vi "AES-InvCipher-BLOCK.vi"(8 "error in (no error)":errorcluster, 10 "Cipher Key":u8[](array[numeric]) format="%02x", 11 "cipher [U8]":u8[](array[numeric]) format="%02x") -> (0 "error out":errorcluster, 3 "plain [U8]":u8[](array[numeric]) format="%02x")   [LabVIEW 2020, in "Encryption.lvlib"]
doc: "Unencrypt a block of U8s that are encrypted with AES.\n\nCAUTION:\nThis VI is not secure, it does not protect the memory of the encryption, key and unencrypted data.\n\n(c) Ton Plomp, 2011\nTHIS SOFTWARE IS PROVIDED AS IS, AND ANY WARRANTY IS REJECTED"
uses:
  Encryption.lvlib
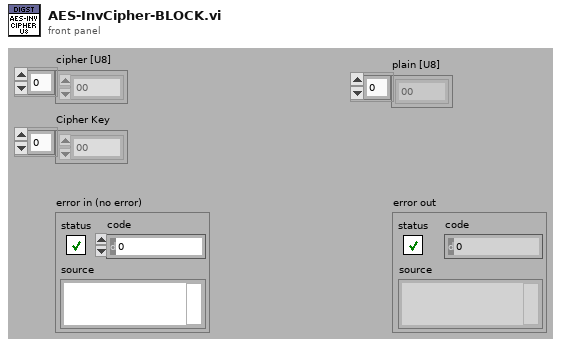
[diagram p1: front panel]
types:
  T1 = cluster{bool, i32, "String to Prepend to source (\"\")":string}
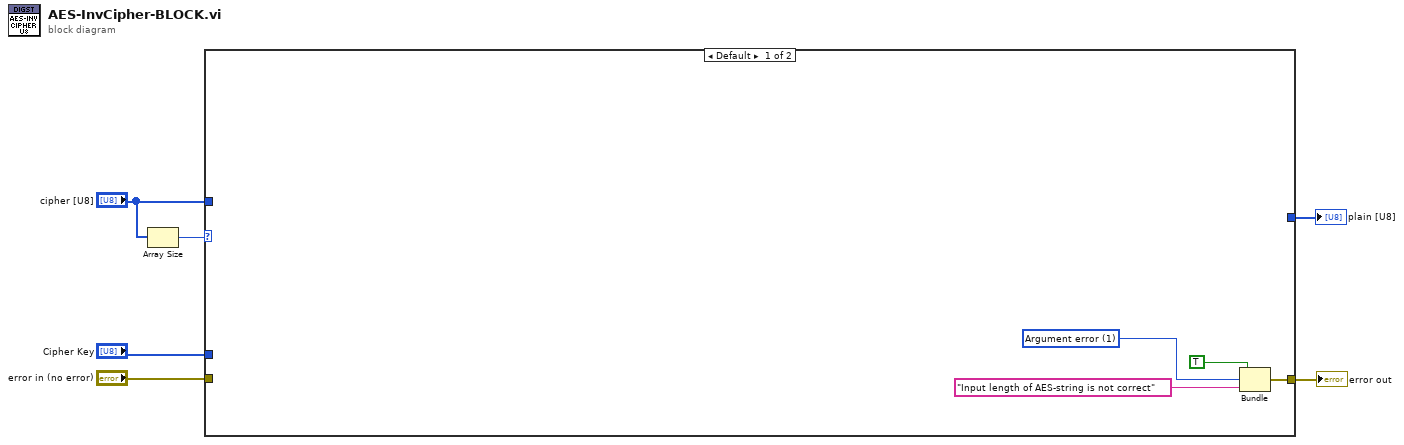
[diagram p0: block diagram]
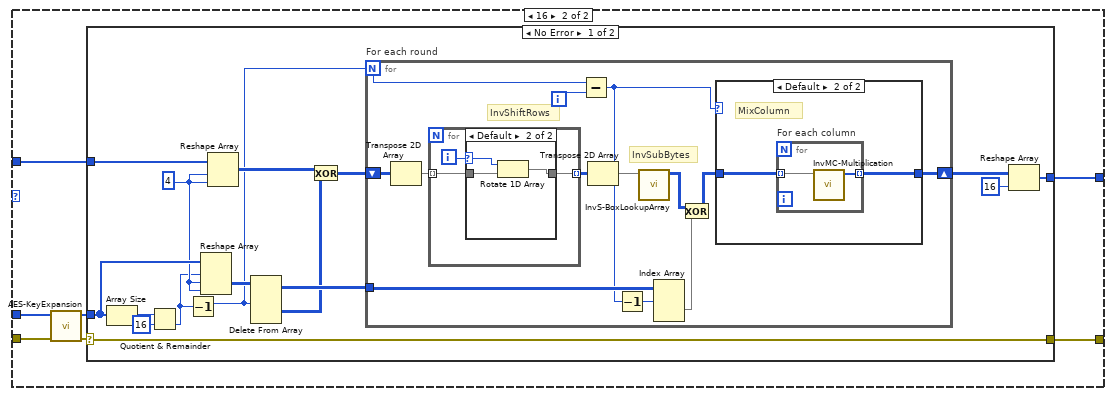
[diagram p2: hidden frame]
diagram:
  n1 = Array Size(array="cipher [U8]") -> (size(s)=w2:i32)
  n2 = case shown="Default" w2 {
    tunnel: [_ w16] -> w6
    tunnel: "Cipher Key" -> [_ w15]
    tunnel: "error in (no error)" -> [_ w14]
    tunnel: "cipher [U8]" -> [_ w13]
    tunnel: [w7 w11] -> w1
    frame Default {
      w8 = 1 items=["No error", "Argument error", "Memory is full", "Out of zone", "End of file", "File already open", "Generic file I/O error", "File not found", "File permission error", "Disk is full", "Duplicate path", "Too many files open", "System feature not enabled", "Resource file not found", "Cannot add resource", "Resource not found", "Image not found", "Image memory error", "Pen does not exist", "Config type invalid", "Config token not found", "Config parse error", "Config memory error", "Bad external code format", "Bad external code offset", "External code not present", "Null window", "Destroy window error", "Null menu", "Print aborted", "Bad print record", "Print driver error", "Windows error during printing", "Memory error during printing", "Print dialog error", "Generic print error", "Invalid device refnum", "Device not found", "Device parameter error", "Device unit error", "Cannot open device", "Device call aborted", "Generic error", "Cancelled by user", "Object ID too low", "Object ID too high", "Object not in heap", "Unknown heap", "Unknown object (invalid DefProc)", "Unknown object (DefProc not in table)", "Message out of range", "Invalid (null) method", "Unknown message", "Manager call not supported", "Bad address", "Network operation in progress", "Network operation timed out", "Connection is busy", "Network attribute not supported", "Network error", "Address in use", "System out of memory", "Connection aborted", "Connection refused", "Not connected", "Already connected", "Connection closed", "Initialization error (interapplication manager)", "Bad occurrence", "Wait on unbound occurrence handler", "Occurrence queue overflow", "Datalog type conflict", "Unused", "Unrecognized type (interapplication manager)", "Memory corrupt", "Failed to make temporary DLL", "Old CIN version", "Drag socket not found", "Failed to load drop-object", "Failed to register OLE object", "Failed to release OLE object", "Format specifier type mismatch", "Unknown format specifier", "Too few format specifiers", "Too many format specifiers", "Scan failed", "Newer CIN version", "Error converting to variant", "Runtime menu error", "Password tampered", "Variant attribute not found", "Incompatible variant data type", "Event data is not available", "Event Store is not present", "Occurrence is not found", "Event Queue is not created", "Event info is not available", "Refnum passed is NULL", "Error retrieving Class GUID", "Error retrieving CoClass GUID", "Error retrieving TypeLib GUID.", "Bad built application magic bytes.", "Specific driver is different from the specific driver associated with the Logical Name.", "There is no session opened to the class driver.", "Max Error", "MAX - Error with config objects", "MAX - Error loading configuration", "MAX - Group not supported"]
      n3 = Bundle(TRUE, w8, "String to Prepend to source (\"\")"="Input length of AES-string is not correct" ("String to Prepend to source (\"\")")) -> (w7:T1)  [unwired: 1 in]
    }
    frame 16 {
      n4 = call "AES-KeyExpansion.vi"("error in (no error)"=w14, "Key In"=w15) -> ("error out"=w12:errorcluster, "Expanded Key [U8]"=w17:u8[])  [unwired: 8 in]
      n5 = case shown="No Error" w12 {
        selector: w12 -> [w22 w59]
        tunnel: w17 -> [w31 _]
        tunnel: [w26 _] -> w16
        tunnel: w13 -> [w24 _]
        tunnel: [w22 w59] -> w11
        frame No Error {
          w23 = 4 ("y")
          n6 = Array Size(array=w31) -> (size(s)=w33:i32)
          n7 = Quotient & Remainder(x=w33, y=16) -> (floor(x/y)=w19:i32)  [unwired: 1 out]
          n8 = Decrement(x=w19) -> (x-1=w18:i32)
          n9 = Reshape Array(w31, w19, w23, w23) -> (w30:u8[][][])
          n10 = Reshape Array(w24, w23, w23) -> (w21:u8[][])
          n11 = Delete From Array(array=w30, index (dim 0)=w18) -> (deleted portion=w20:u8[][], array with subset deleted=w29:u8[][][])  [unwired: 3 in]
          n12 = Exclusive Or(1:w20, 2:w21) -> (0:w28:u8[][])
          n13 = for "For each round" {
            N: w18 -> [w46]
            shift-right: [w34] -> w27
            shift-left: w28 -> [w44]
            tunnel: w29 -> [w39]
            i -> [w45]
            # "InvShiftRows"
            # "InvSubBytes"
            n14 = Transpose 2D Array(2D array=w44) -> (transposed array=w42:u8[][])
            n15 = for {
              tunnel: w42 -> [w53] mode=indexing
              tunnel: [w52] -> w43 mode=indexing
              i -> [w54]
              n16 = case shown="Default" w54 {
                selector: w54 -> [_ w56]
                tunnel: w53 -> [w55 w58]
                tunnel: [w55 w57] -> w52
                frame 0 {
                }
                frame Default {
                  n17 = Rotate 1D Array(1:w58, 2:w56) -> (0:w57:u8[])
                }
              }
            }
            n18 = Subtract(x=w46, y=w45) -> (x-y=w38:i32)
            n19 = Transpose 2D Array(2D array=w43) -> (transposed array=w41:u8[][])
            n20 = Decrement(x=w38) -> (x-1=w37:i32)
            n21 = call "InvS-BoxLookupArray.vi"("In"=w41) -> ("Out"=w40:u8[][])  [unwired: 10 in]
            n22 = Index Array(array=w39, index (dim 0)=w37) -> (element=w36:u8[][])  [unwired: 2 in]
            n23 = Exclusive Or(1:w36, 2:w40) -> (0:w35:u8[][])
            n24 = case shown="Default" w38 {
              tunnel: w35 -> [w47 w49]
              tunnel: [w47 w48] -> w34
              frame 1 {
                # "Last Round"
              }
              frame Default {
                # "MixColumn"
                n25 = for "For each column" {
                  tunnel: w49 -> [w50] mode=indexing
                  tunnel: [w51] -> w48 mode=indexing
                  n26 = call "InvMC-Multiplication.vi"("Vector In"=w50) -> ("Vector Out"=w51:u8[])  [unwired: 10 in]
                }
              }
            }
          }
          n27 = Reshape Array(w27, 16 ("dimension size")) -> (w26:u8[])
        }
        frame Error {
        }
      }
    }
  }
  "error out" <- w1
  "plain [U8]" <- w6
